vi "Test_WriteMixedTypes_ReadNoFilter_ReturnAll.vi"(8 "error in (no error)":errorcluster, 11 "TestCase in":refnum<class "TestComposedLookupTable.lvclass">) -> (0 "error out":errorcluster, 3 "TestCase out":refnum<class "TestComposedLookupTable.lvclass">)   [LabVIEW 2017, in "TestComposedLookupTable.lvclass"]
uses:
  TestComposedLookupTable.lvclass
  Source/LookupTable/LookupTable.lvclass/LookupTable.ctl
  427e9736-e78b-429d-97ac-30c52520a778.vi
  ce18b910-b9e6-47ff-9f46-5f252a51b4d1.vi
  582381f8-cc50-42f8-acca-1be279f157b5.vi
  a55ae4b1-3c32-4eb4-b263-9ff7262b8e90.vi
  Source/LookupTable/Read Table Reference.vi
  427e9736-e78b-429d-97ac-30c52520a778.vi/773f923d-4a18-40cc-9f7e-3161ac70a1d1.vi
  ce18b910-b9e6-47ff-9f46-5f252a51b4d1.vi/4ced25cf-c1c3-4ce6-9cf4-819b249cf6e0.vi
  582381f8-cc50-42f8-acca-1be279f157b5.vi/fa7b6a64-7c6f-4ae1-8aab-9f7b19700e69.vi
  Source/LookupTable/LookupTable.lvclass
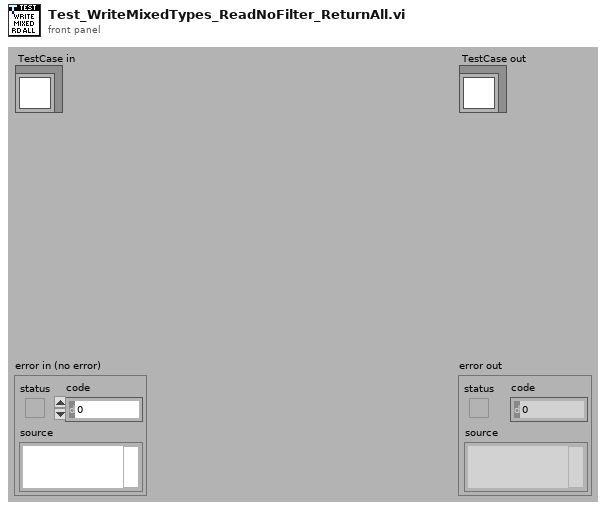
[diagram p1: front panel]
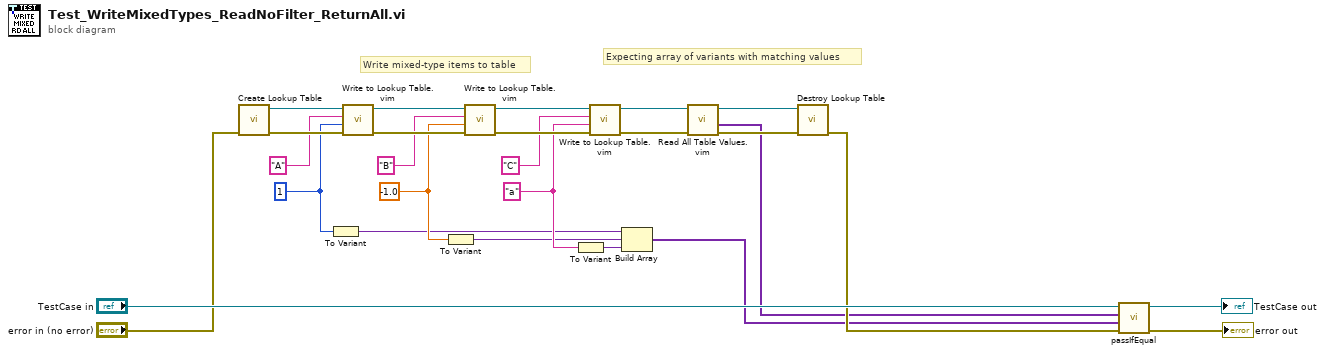
[diagram p0: block diagram]
diagram:
  w5 = "a"
  w6 = -1.0
  w7 = 1
  # "Expecting array of variants with matching values"
  # "Write mixed-type items to table"
  n1 = call "Create Lookup Table.vi"("error in (no error)"="error in (no error)") -> ("error out"=w25:errorcluster, "LookupTable Reference"=w18:refnum<data-value>)  [unwired: 9 in]
  n2 = To Variant(anything=w7) -> (Variant=w4:variant)
  n3 = call "Write to Lookup Table.vim"("error in (no error)"=w25, "Item"=w7, "Item Name"="A", "LookupTable Reference"=w18) -> ("error out"=w20:errorcluster, "LookupTable Reference Out"=w21:refnum<data-value>)  [unwired: 5 in, 1 out]
  n4 = To Variant(anything=w6) -> (Variant=w3:variant)
  n5 = call "Write to Lookup Table.vim"("error in (no error)"=w20, "Item"=w6, "Item Name"="B", "LookupTable Reference"=w21) -> ("error out"=w26:errorcluster, "LookupTable Reference Out"=w13:refnum<data-value>)  [unwired: 5 in, 1 out]
  n6 = To Variant(anything=w5) -> (Variant=w2:variant)
  n7 = call "Write to Lookup Table.vim"("error in (no error)"=w26, "Item"=w5, "Item Name"="C", "LookupTable Reference"=w13) -> ("error out"=w12:errorcluster, "LookupTable Reference Out"=w10:refnum<data-value>)  [unwired: 5 in, 1 out]
  n8 = Build Array(w4, w3, w2) -> (w1:variant[])
  n9 = call "Read All Table Values.vim"("error in (no error)"=w12, "LookupTable Reference"=w10) -> ("error out"=w11:errorcluster, "Values"=w8:variant[], "LookupTable Reference Out"=w9:refnum<data-value>)  [unwired: 6 in, 1 out]
  n10 = call "Destroy Lookup Table.vi"("error in (no error)"=w11, "LookupTable Reference"=w9) -> ("error out"=w16:errorcluster)  [unwired: 9 in]
  n11 = call-dynamic "passIfEqual.vi"("error in (no error)"=w16, "y"=w1, "x"=w8, "TestCase in"="TestCase in") -> ("error out"=→"error out":errorcluster, "TestCase out"=→"TestCase out":refnum<class "TestComposedLookupTable.lvclass">)  [unwired: 6 in]
